vi "Write Startup Launch Nested Views Msg.vi"(10 "Launch Nested Views Msg":refnum<class "Launch Nested Views Msg.lvclass">, 11 "Popup ViewManager in":refnum<class "Popup ViewManager.lvclass">) -> (3 "Popup ViewManager out":refnum<class "Popup ViewManager.lvclass">)   [LabVIEW 2020, in "Popup ViewManager.lvlib" / "Popup ViewManager.lvclass"]
uses:
  <vilib>/gpm_packages/@cs/popup-viewmanager/Source/Popup ViewManager/Popup ViewManager.lvclass
  <vilib>/gpm_packages/@cs/popup-viewmanager/Source/Popup ViewManager Messages/Launch Nested Views Msg/Launch Nested Views Msg.lvclass
  <vilib>/gpm_packages/@cs/popup-viewmanager/Source/Popup ViewManager/Popup ViewManager.lvclass/Popup ViewManager.ctl
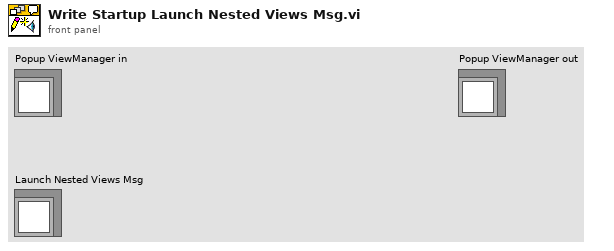
[diagram p1: front panel]
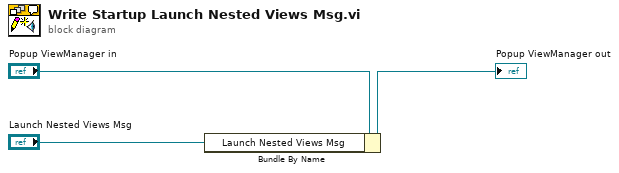
[diagram p0: block diagram]
diagram:
  n1 = Bundle By Name(cluster="Popup ViewManager in", "Launch Nested Views Msg"="Launch Nested Views Msg") -> (→"Popup ViewManager out":refnum<class "Popup ViewManager.lvclass">)
